vi "Exemple_Extraction_Patches_2D.vi"() -> ()   [LabVIEW 2020]
panel:
  out "Data":T1
  in  "Image":u16(ring) items=["China", "Flower"]
  in  "extract_patches_2d":T2={"patch_size"={"patch_height"=2, "patch_width"=2}, "max_patches"="None", "random_state"=-1} {"random_state" min=-1}
  out "error out":errorcluster caption="sortie d'erreur"
  in  "error in":errorcluster caption="entrée d'erreur"
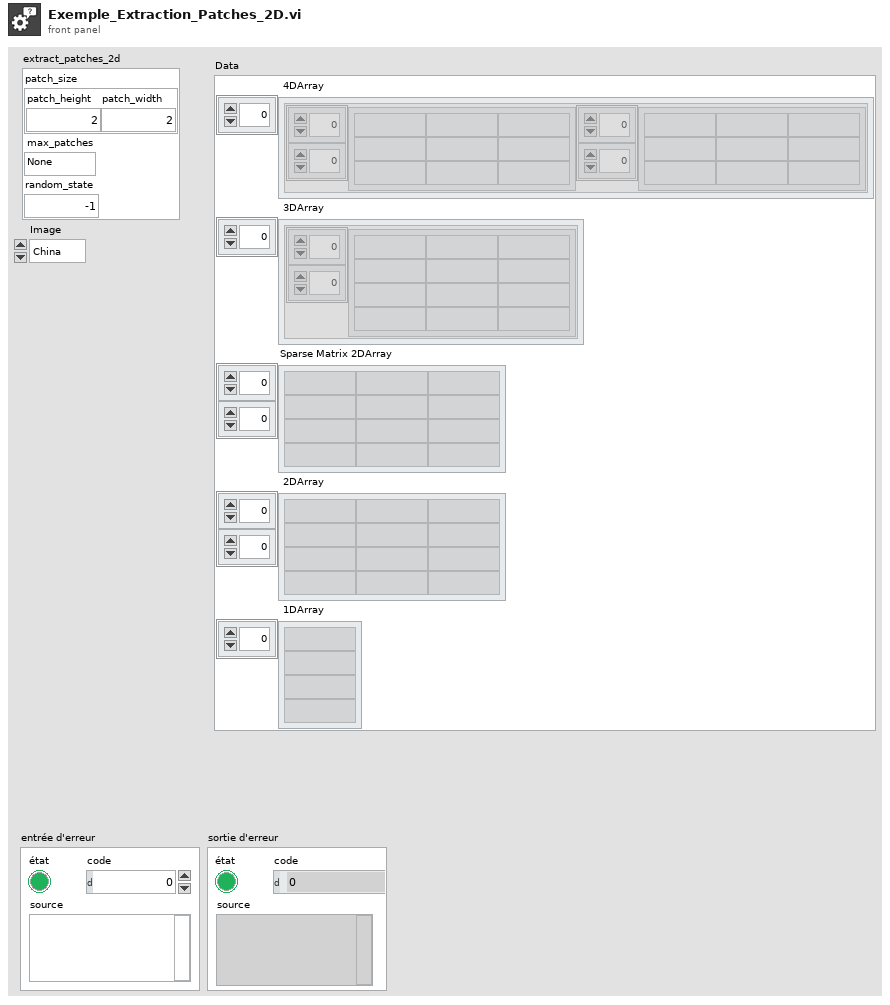
[diagram p1: front panel]
types:
  T1 = cluster{" 4DArray":cluster{"1":string[][], "2":string[][]}[], " 3DArray":cluster{"Tableau":string[][]}[], "Sparse Matrix 2DArray":string[][], " 2DArray":string[][], " 1DArray":string[]}
  T2 = cluster{"patch_size":cluster{"patch_height":i32, "patch_width":i32}, "max_patches":string, "random_state":i32}
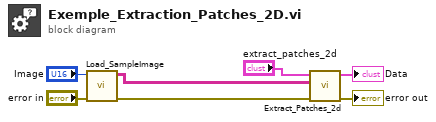
[diagram p0: block diagram]
diagram:
  n1 = call "Load_SampleImage.vi"("error in"="error in", "Image"="Image") -> ("error out"=w5:errorcluster, "Image (RGB)"=w3:string[][])  [unwired: 8 in]
  n2 = call "Extract_Patches_2d.vi"("error in"=w5, "Image"=w3, "extract_patches_2d"="extract_patches_2d") -> ("error out"=→"error out":errorcluster, "Data"=→"Data":T1)  [unwired: 7 in]
